vi "KE22XX_Supply_Off_all_Channels.vi"(0 "Supply_1":refnum<visa-resource-name>="COM32", 5 "Supply_2":refnum<visa-resource-name>="COM20", 11 "Error In":errorcluster, 12 "Channe 1":T1={"Output ?"=FALSE, "Enable"=TRUE, "Voltage Level (V)"=1.5, "Current Limit (A) "=0.01}, 13 "Channe 2":T1={"Output ?"=FALSE, "Enable"=TRUE, "Voltage Level (V)"=1.35, "Current Limit (A) "=0.01}, 14 "Channe 3":T1={"Output ?"=FALSE, "Enable"=TRUE, "Voltage Level (V)"=3.3, "Current Limit (A) "=0.02}) -> (15 "error out":errorcluster)   [LabVIEW 2016]
uses:
  Channel Control.ctl
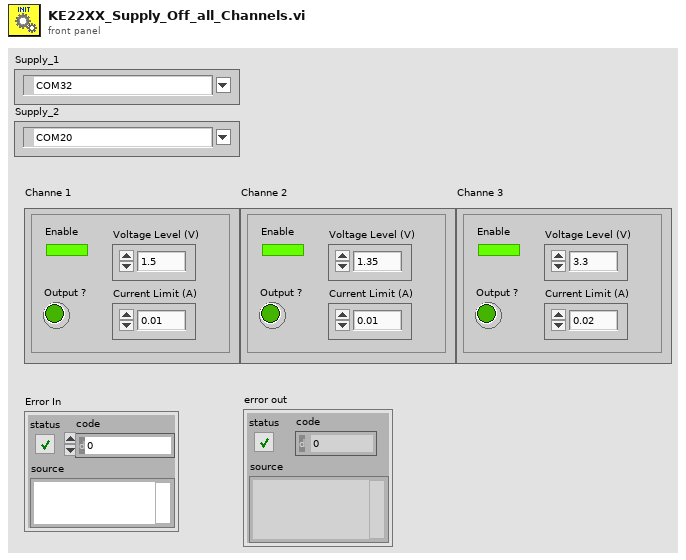
[diagram p1: front panel]
types:
  T1 = typedef "Channel Control.ctl" = cluster{"Output ?":bool, "Enable":bool, "Voltage Level (V)":dbl, "Current Limit (A) ":dbl}
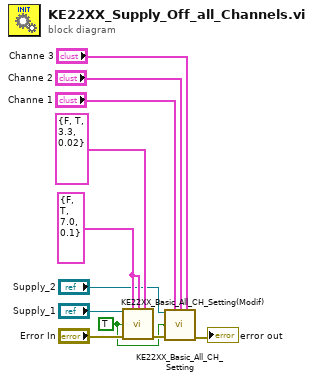
[diagram p0: block diagram]
diagram:
  w5 = TRUE ("Remote")
  w8 = T1 {"Output ?"=FALSE, "Enable"=TRUE, "Voltage Level (V)"=7.0, "Current Limit (A) "=0.1} ("Channe 1")
  n1 = call "KE22XX_Basic_All_CH_Setting(Modif).vi"("VISA In"="Supply_1", "Channe 1"=w8, "Channe 2"=w8, "Channe 3"=T1 {"Output ?"=FALSE, "Enable"=TRUE, "Voltage Level (V)"=3.3, "Current Limit (A) "=0.02} ("Channe 1"), "Remote"=w5, "error in"="Error In") -> ("error out"=w10:errorcluster)  [unwired: 9 in]
  n2 = call "KE22XX_Basic_All_CH_Setting.vi"("VISA In"="Supply_2", "Channe 1"="Channe 1", "Channe 2"="Channe 2", "Channe 3"="Channe 3", "Remote"=w5, "error in"=w10) -> ("error out"=→"error out":errorcluster)  [unwired: 9 in]
